vi "ReadWriteServiceRequest.vi"(4 "Service ROS":T2={"topic port"=1236, "Node"="/labview", "topic"="/robot/head/command_head_nod", "type"="std_msgs/Bool", "node port"=7000, "error "={"status"=FALSE, "code"=0, "source"=""}, "Direction"=enum."Publisher", "APIs"=[], "Update (ms)"=1, "write queue"=1}, 5 "Error in":path, 6 "data":string, 7 "Log in":T4[](array[typedef])) -> (0 "Error out":path, 1 "String Read":string, 2 "Log":T4[](array[typedef]), 3 "MyState":T5)   [LabVIEW 2012]
uses:
  <userlib>/ROSforLV/ROS/Code/Console/Servers/ServerSubs/MyState.ctl
  <userlib>/ROSforLV/ROS/Code/Console/Servers/ServerSubs/ROSLog.ctl
  <userlib>/ROSforLV/ROS/Code/SubVIs/_ROSControl.ctl
  <userlib>/ROSforLV/ROS/Code/SubVIs/_ROSDirection.ctl
panel:
  out "Connections":T1(array[cluster])
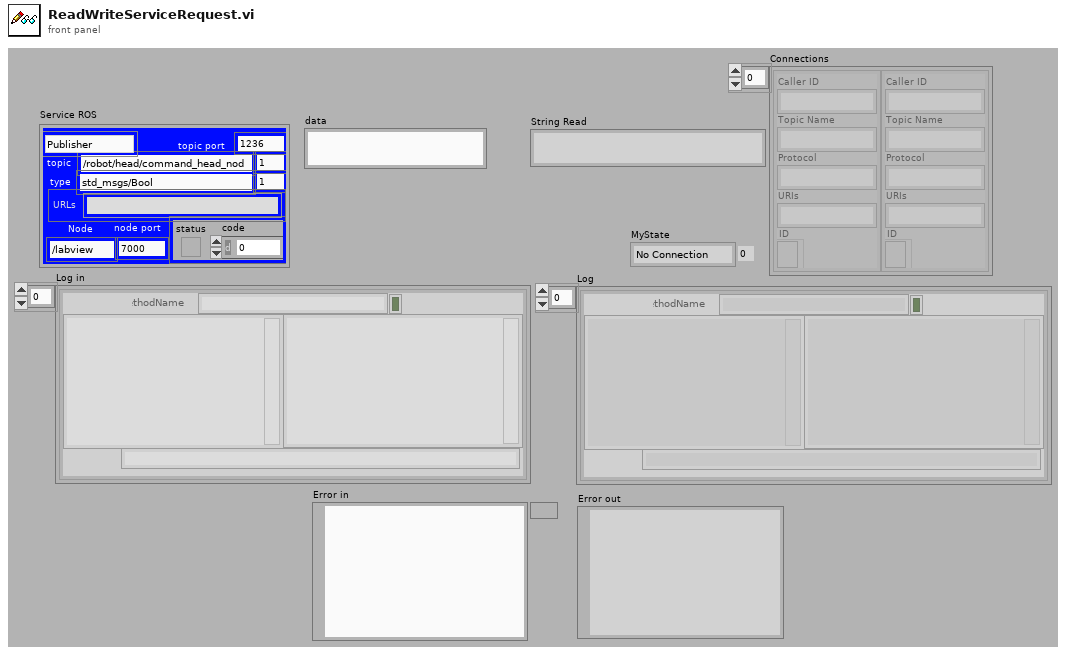
[diagram p1: front panel]
types:
  T1 = cluster{"Caller ID":string, "Topic Name":string, "Protocol":string, "URIs":string, "ID":refnum<k5>}[]
  T2 = typedef "_ROSControl.ctl" = cluster{"topic port":u16, "Node":string, "topic":string, "type":string, "node port":u32, "error ":errorcluster, "Direction":T3, "APIs":string[], "Update (ms)":u16, "write queue":u16}
  T3 = typedef "_ROSDirection.ctl" = enum16{"Node", "Publisher", "Subscriber", "Service Client"}
  T4 = typedef "ROSLog.ctl" = cluster{"Sent":string, "Reply":string, "MethodName":string, "success":bool, "Dir1":string, "Dir2":string, "Time Stamp":string, "error":errorcluster, "Preamble":string}
  T5 = typedef "MyState.ctl" = enum16{"No Connection", "Registered", "Connected", "Close"}
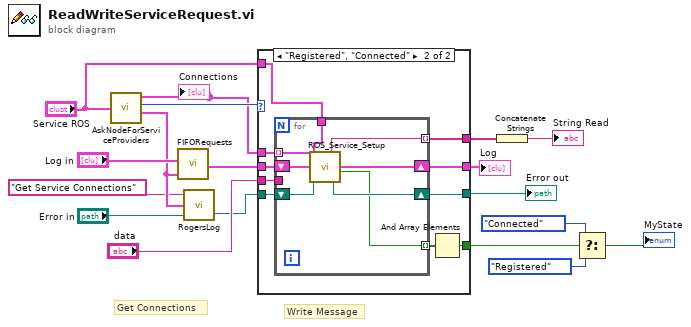
[diagram p0: block diagram]
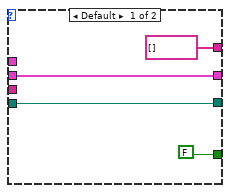
[diagram p2: hidden frame]
diagram:
  # "Write Message"
  # "Get Connections"
  n1 = call <userlib>:"AskNodeForServiceProviders.vi"("Service ROS"="Service ROS") -> ("Connections"=w8:T1, "MyState"=w13:T5, "Log"=w4:T4)  [unwired: 1 in]
  "Connections" <- w8
  n2 = call <userlib>:"FIFORequests.vi"("Log"=w4, "Requests in"="Log in") -> ("Requests out"=w14:T4[])  [unwired: 1 in]
  n3 = call <userlib>:"RogersLog.vi"("Text to add"="Get Service Connections", "Log"=w4, "LogPath in"="Error in") -> ("LogPath out"=w2:path)  [unwired: 2 in, 1 out]
  n4 = case shown="\"Registered\", \"Connected\"" w13 {
    tunnel: [w19 w28] -> w1
    tunnel: "data" -> [_ w32]
    tunnel: [w22 w30] -> w9
    tunnel: w8 -> [_ w29]
    tunnel: w14 -> [w22 w31]
    tunnel: [string[] [] w27] -> w12
    tunnel: [FALSE ("status") w25] -> w7
    tunnel: "Service ROS" -> [_ w24]
    tunnel: w2 -> [w19 w23]
    frame Default {
    }
    frame "Registered", "Connected" {
      n5 = for {
        tunnel: w32 -> [_]
        shift-right: [w39] -> w30
        shift-left: w31 -> [w40]
        tunnel: w24 -> [w38]
        tunnel: w29 -> [w37] mode=indexing
        shift-right: [w34] -> w28
        shift-left: w23 -> [w35]
        tunnel: [w36] -> w27 mode=indexing
        tunnel: [w33] -> w26 mode=indexing
        n6 = call <userlib>:"ROS_Service_Setup.vi"("Subscriber"=w37, 6:"Log in"=w35, "ROS"=w38, 8:"Log in"=w40) -> (0:"Log out"=w34:path, "Success?"=w33:bool, "Reply"=w36:string, 3:"Log out"=w39:T4[])  [unwired: 1 in]
      }
      n7 = And Array Elements(Boolean array=w26) -> (logical AND=w25:bool)
    }
  }
  "Error out" <- w1
  "Log" <- w9
  n8 = Concatenate Strings(w12) -> (→"String Read":string)
  n9 = Select(t=MyState."Connected" ("MyState"), s=w7, f=MyState."Registered" ("MyState")) -> (s? t:f=→"MyState":T5)
